vi "Load Components.vi"(8 "error in (no error)":errorcluster, 10 "component names":string[](array[string]), 11 "Component Loader in":refnum<class "Component Loader.lvclass">) -> (0 "error out":errorcluster, 2 "component objects":refnum<class>[](array[class]), 3 "Component Loader out":refnum<class "Component Loader.lvclass">)   [LabVIEW 2017, in "DSF Core.lvlib" / "Component Loader.lvclass"]
uses:
  Component Loader.lvclass
  Components/Transceivers/UDP/DSF UDP Transceiver.lvclass
  Components/Buffer Converters/DSF Type Converter/DSF Buffer Converter.lvclass
  DSF Core.lvlib
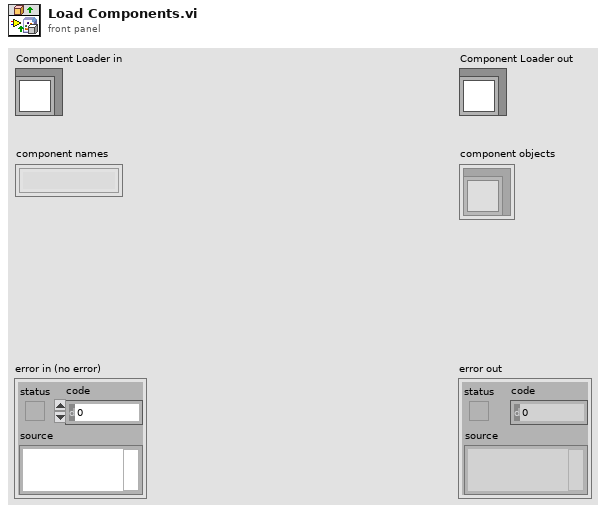
[diagram p1: front panel]
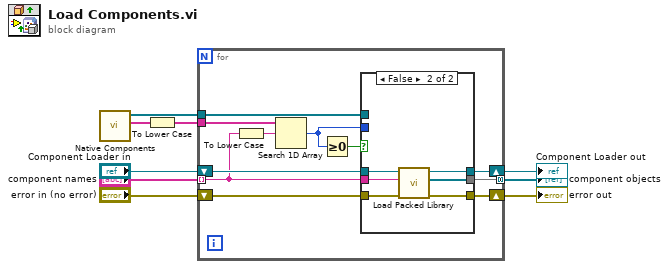
[diagram p0: block diagram]
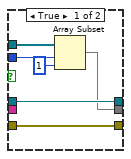
[diagram p2: hidden frame]
diagram:
  n1 = call "Native Components.vi"() -> ("native component names"=w3:string[], "native component objects"=w2:refnum<class>[])  [unwired: 9 in, 1 out]
  n2 = To Lower Case(string=w3) -> (all lower case string=w1:string[])
  n3 = for {
    shift-right: [w17] -> w6
    shift-left: "Component Loader in" -> [w20]
    shift-right: [w18] -> w5
    shift-left: "error in (no error)" -> [w19]
    tunnel: [w16] -> w7 mode=concatenating
    tunnel: "component names" -> [w14] mode=indexing
    tunnel: w1 -> [w15]
    tunnel: w2 -> [w12]
    n4 = To Lower Case(string=w14) -> (all lower case string=w10:string)
    n5 = Search 1D Array(1D array=w15, element=w10) -> (index of element=w11:i32)  [unwired: 1 in]
    n6 = Greater Or Equal To 0?(x=w11) -> (x >= 0?=w13:bool)
    n7 = case shown="False" w13 {
      tunnel: w20 -> [w26 w32]
      tunnel: w19 -> [w25 w31]
      tunnel: [w25 w30] -> w18
      tunnel: [w26 w29] -> w17
      tunnel: [w21 w28] -> w16
      tunnel: w14 -> [_ w27]
      tunnel: w12 -> [w24 _]
      tunnel: w11 -> [w22 _]
      frame True {
        n8 = Array Subset(array=w24, index=w22, length=1) -> (w21:refnum<class>[])
      }
      frame False {
        n9 = call "Load Packed Library.vi"("error in (no error)"=w31, "packed library name"=w27, "Component Loader in"=w32) -> ("error out"=w30:errorcluster, "objects"=w28:refnum<class>[], "Component Loader out"=w29:refnum<class "Component Loader.lvclass">)  [unwired: 6 in]
      }
    }
  }
  "error out" <- w5
  "Component Loader out" <- w6
  "component objects" <- w7
